vi "Call (async) MsgPack.vi"(4 "ArgumentsKw":refnum<class "MsgPackMap.lvclass">, 6 "Arguments":refnum<class "MsgPackArray.lvclass">, 7 "Options":refnum<class "MsgPackMap.lvclass">, 8 "error in (no error)":errorcluster, 9 "Notify result":bool, 10 "Topic URI":string, 11 "WAMP Client in":refnum<class "WAMP Client.lvclass">) -> (0 "error out":errorcluster, 2 "Call result notifier":refnum<notifier>, 3 "WAMP Client out":refnum<class "WAMP Client.lvclass">)   [LabVIEW 2020, in "wamplv.lvlib" / "WAMP Client.lvclass"]
uses:
  WAMP Client.lvclass
  MessagePack/MsgPackArray/MsgPackArray.lvclass
  MessagePack/MsgPackMap/MsgPackMap.lvclass
  TypeDefs/RESULT payload (MsgPack).ctl
  TypeDefs/Combined error.ctl
  TypeDefs/WAMP error.ctl
  TypeDefs/Serialisation.ctl
  WAMP Client.lvclass/WAMP Client.ctl
  Private/TypeDefs/CALL request (MsgPack).ctl
  Private/TypeDef/Internal Message Type.ctl
  44dd0fb6-e4b1-424e-8704-d5c62803e1d5.vi
  Is Connected.vi
  Private/SubVIs/Matches serialisation type.vi
  <vilib>/Utility/error.llb/Error Cluster From Error Code.vi
  Private/SubVIs/Check URI.vi
  wamplv.lvlib
  Private/Requests/CallRequest (MsgPack)/CallRequest (MsgPack).lvclass
  C:/local/wamplv/Private/Requests/CallRequest (MsgPack)/CallRequest (MsgPack).lvclass
  C:/local/wamplv/Private/Requests/ICallRequest/ICallRequest.lvclass
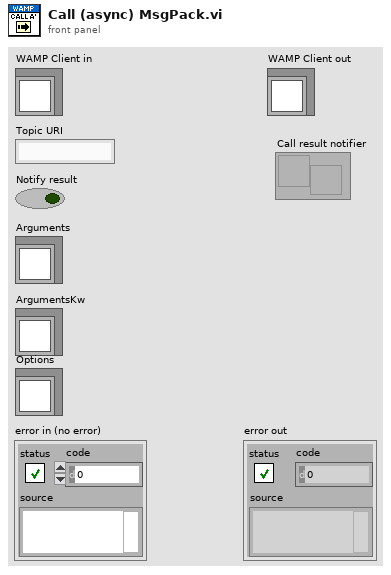
[diagram p1: front panel]
types:
  T1 = typedef "wamplv.lvlib/WAMP Client.lvclass/Serialisation.ctl" = enum16{"JSON", "MessagePack"}
  T2 = typedef "wamplv.lvlib/WAMP Client.lvclass/RESULT payload (MsgPack).ctl" = cluster{"Topic":string, "Arguments Payload":refnum<class "MsgPackArray.lvclass">, "ArgumentKw Payload":refnum<class "MsgPackMap.lvclass">, "Combined Error":T3}
  T3 = typedef "wamplv.lvlib/WAMP Client.lvclass/Combined error.ctl" = cluster{"Error?":bool, "WAMP Error":T4, "Error":errorcluster}
  T4 = typedef "wamplv.lvlib/WAMP Client.lvclass/WAMP error.ctl" = cluster{"Details":string, "ArgumentKw Payload":string, "Error?":bool, "Error URI":string, "Arguments Payload":string}
  T5 = typedef "wamplv.lvlib/CALL request (MsgPack).ctl" = cluster{"Topic URI":string, "Arguments":refnum<class "MsgPackArray.lvclass">, "ArgumentsKw":refnum<class "MsgPackMap.lvclass">, "Options":refnum<class "MsgPackMap.lvclass">, "Call Result":refnum<notifier>}
  T6 = typedef "wamplv.lvlib/WAMP Client.lvclass/Internal Message Type.ctl" = enum16{"Subscribe", "Handle Subscribed", "Handle Event", "Unsubscribe", "Handle Unsubscribed", "Publish", "Handled Published", "Goodbye", "Handle Goodbye", "Call", "Handle Result", "Register", "Handle Registered", "Unregister", "Handle Unregistered", "Handle Invocation", "Yield", "Error"}
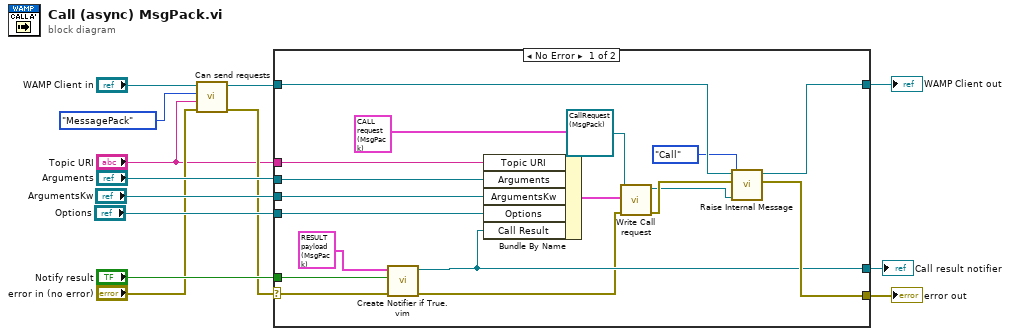
[diagram p0: block diagram]
diagram:
  n1 = call "Can send requests.vi"("error in (no error)"="error in (no error)", "Topic URI"="Topic URI", "Serialisation"=Serialisation."MessagePack", "WAMP Client in"="WAMP Client in") -> ("error out"=w5:errorcluster, "WAMP Client out"=w6:refnum<class "WAMP Client.lvclass">)  [unwired: 6 in]
  n2 = case shown="No Error" w5 {
    selector: w5 -> [w23 w33]
    tunnel: [w28 w33] -> w13
    tunnel: [w30 w32] -> w12
    tunnel: w6 -> [w31 w32]
    tunnel: "Topic URI" -> [w27 _]
    tunnel: "Arguments" -> [w26 _]
    tunnel: "ArgumentsKw" -> [w25 _]
    tunnel: "Options" -> [w24 _]
    tunnel: [w19 _] -> w7
    tunnel: "Notify result" -> [w22 _]
    frame No Error {
      n3 = call "Create Notifier if True.vim"("error in (no error)"=w23, "Boolean"=w22, "RESULT Payload"=T2 {"Topic"="", "Arguments Payload"=refnum, "ArgumentKw Payload"=refnum, "Combined Error"={"Error?"=FALSE, "WAMP Error"={"Details"="{}", "ArgumentKw Payload"="{}", "Error?"=FALSE, "Error URI"="", "Arguments Payload"=""}, "Error"={"status"=FALSE, "code"=0, "source"=""}}}) -> ("error out"=w16:errorcluster, "Notifier out"=w19:refnum<notifier>)  [unwired: 7 in]
      n4 = Bundle By Name(cluster=T5 {"Topic URI"="", "Arguments"=refnum, "ArgumentsKw"=refnum, "Options"=refnum, "Call Result"=refnum} ("Cluster"), "Topic URI"=w27, "Arguments"=w26, "ArgumentsKw"=w25, "Options"=w24, "Call Result"=w19) -> (w18:T5)
      n5 = call "Write Call request.vi"("error in (no error)"=w16, "Cluster"=w18, "CallRequest (MsgPack) in"=refnum<class "CallRequest (MsgPack).lvclass"> refnum) -> ("error out"=w15:errorcluster, "CallRequest (MsgPack) out"=w14:refnum<class "CallRequest (MsgPack).lvclass">)  [unwired: 7 in]
      n6 = call "Raise Internal Message.vi"("Variant"=w14, "Internal Message Type"=Internal_Message_Type."Call", "error in (no error)"=w15, "WAMP Client in"=w31) -> ("error out"=w28:errorcluster, "WAMP Client out"=w30:refnum<class "WAMP Client.lvclass">)  [unwired: 6 in]
    }
    frame Error {
    }
  }
  "error out" <- w13
  "WAMP Client out" <- w12
  "Call result notifier" <- w7
